vi "Debug_Convert_Data_to_String.vi"(8 "error in (no error)":errorcluster, 11 "AB_Source_Exported_Assembly_VI in":refnum<class "AB_Source_Exported_Assembly_VI.lvclass">) -> (0 "error out":errorcluster, 1 "classData":string, 2 "sourceType":string, 3 "AB_Source_Exported_Assembly_VI out":refnum<class "AB_Source_Exported_Assembly_VI.lvclass">)   [LabVIEW 2020, in "AB_Source_Exported_Assembly_VI.lvclass"]
uses:
  <vilib>/AppBuilder/AB_Classes/Source/ExportedAssemblyVI/AB_Source_Exported_Assembly_VI.lvclass
  <vilib>/AppBuilder/AB_Classes/Source/ExportedAssemblyVI/AB_Source_Exported_Assembly_VI.lvclass/AB_Source_Exported_Assembly_VI.ctl
  <vilib>/AppBuilder/AB_Classes/Source/VI/AB_Source_VI.lvclass
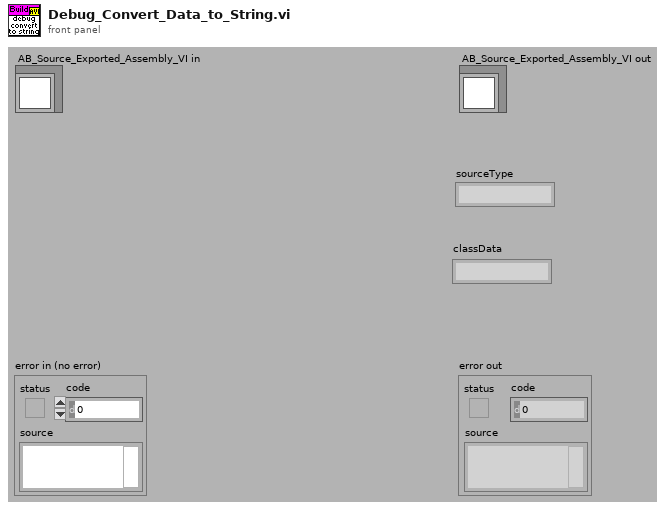
[diagram p1: front panel]
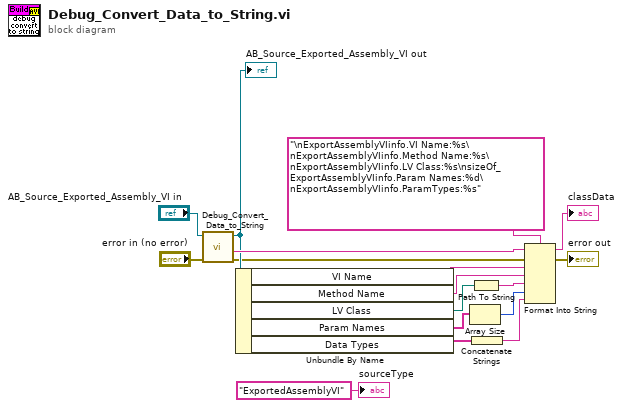
[diagram p0: block diagram]
diagram:
  n1 = call-parent "Debug_Convert_Data_to_String.vi"("error in (no error)"="error in (no error)", "AB_Source_VI in"="AB_Source_Exported_Assembly_VI in") -> ("error out"=w2:errorcluster, "classData"=w13:string, "AB_Source_VI out"=w12:refnum<class "AB_Source_Exported_Assembly_VI.lvclass">)  [unwired: 7 out]
  "AB_Source_Exported_Assembly_VI out" <- w12
  n2 = Unbundle By Name(w12) -> ("VI Name"=w14:string, "Method Name"=w11:string, "LV Class"=w10:path, "Param Names"=w4:string[], "Data Types"=w6:string[])
  n3 = Array Size(array=w4) -> (size(s)=w3:i32)
  n4 = Path To String(path=w10) -> (string=w9:string)
  n5 = Concatenate Strings(w6) -> (w5:string)
  n6 = Format Into String(format string="\nExportAssemblyVIinfo.VI Name:%s\nExportAssemblyVIinfo.Method Name:%s\nExportAssemblyVIinfo.LV Class:%s\nsizeOf_ExportAssemblyVIinfo.Param Names:%d\nExportAssemblyVIinfo.ParamTypes:%s", initial string=w13, error in=w2, w14, w11, w9, w3, w5) -> (resulting string=→"classData":string, error out=→"error out":errorcluster)
  "sourceType" <- "ExportedAssemblyVI" ("sourceType")
